vi "Cluster - Get Result.vi"(8 "error in (no error)":errorcluster, 11 "Cluster With Class":T1) -> (0 "error out":errorcluster, 2 "Result":dbl, 3 "Cluster With Class Out":T1)   [LabVIEW 2010]
uses:
  ClassDefinitions/SimpleClassWithMethods/SimpleArithmetic.lvclass
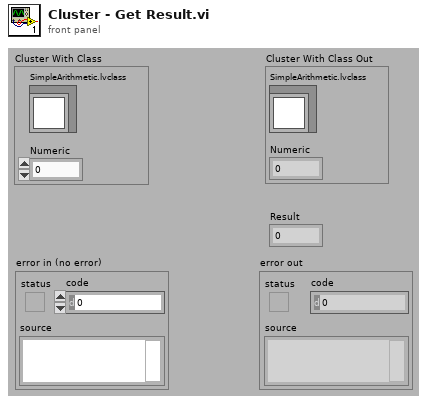
[diagram p1: front panel]
types:
  T1 = cluster{"SimpleArithmetic.lvclass":refnum<class "SimpleArithmetic.lvclass">, "Numeric":dbl}
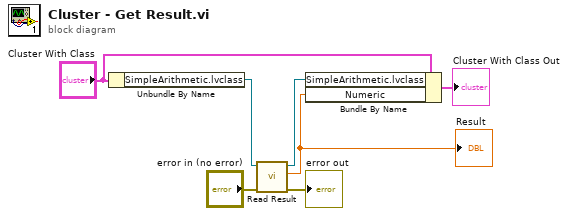
[diagram p0: block diagram]
diagram:
  n1 = Unbundle By Name("Cluster With Class") -> ("SimpleArithmetic.lvclass"=w7:refnum<class "SimpleArithmetic.lvclass">)
  n2 = call "Read Result.vi"("error in (no error)"="error in (no error)", "SimpleArithmetic in"=w7) -> ("error out"=→"error out":errorcluster, "Result"=w1:dbl, "SimpleArithmetic out"=w6:refnum<class "SimpleArithmetic.lvclass">)  [unwired: 7 in]
  "Result" <- w1
  n3 = Bundle By Name(cluster="Cluster With Class", "SimpleArithmetic.lvclass"=w6, "Numeric"=w1) -> (→"Cluster With Class Out":T1)
